vi "Excel - Open Docuement Tests.vi"(8 "error in (no error)":errorcluster) -> (0 "error out":errorcluster)   [LabVIEW 2020]
uses:
  src/LabVIEW NPOI/MS-Excel/MS-Excel.lvclass
  D:/Benjamin/Documents/Perso/Code/WC/LabVIEW_NPOI/src/LabVIEW NPOI/Document/Document.lvclass
  src/LabVIEW NPOI/MS-Excel/Get Workbook.vi
  <vilib>/addons/_JKI Toolkits/Caraya/classes/Assert/Assert Not Error.vi
  <vilib>/addons/_JKI Toolkits/Caraya/classes/Assert/Assert False.vi
  <vilib>/addons/_JKI Toolkits/Caraya/classes/Assert/Assert Error.vi
  <vilib>/addons/_JKI Toolkits/Caraya/classes/Assert/Assert True.vi
  D:/Benjamin/Documents/Perso/Code/WC/LabVIEW_NPOI/lib/NPOI 2.1.1/NPOI.dll
  lib/NPOI 2.1.1/NPOI.dll
  src/LabVIEW NPOI/Document/Document.lvclass
  <vilib>/addons/_JKI Toolkits/Caraya/classes/Test/Test.lvclass
  <vilib>/addons/_JKI Toolkits/Caraya/classes/Assert/Assert.lvclass
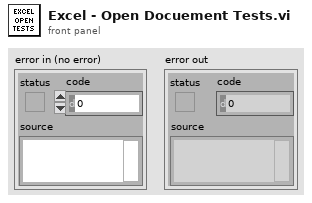
[diagram p1: front panel]
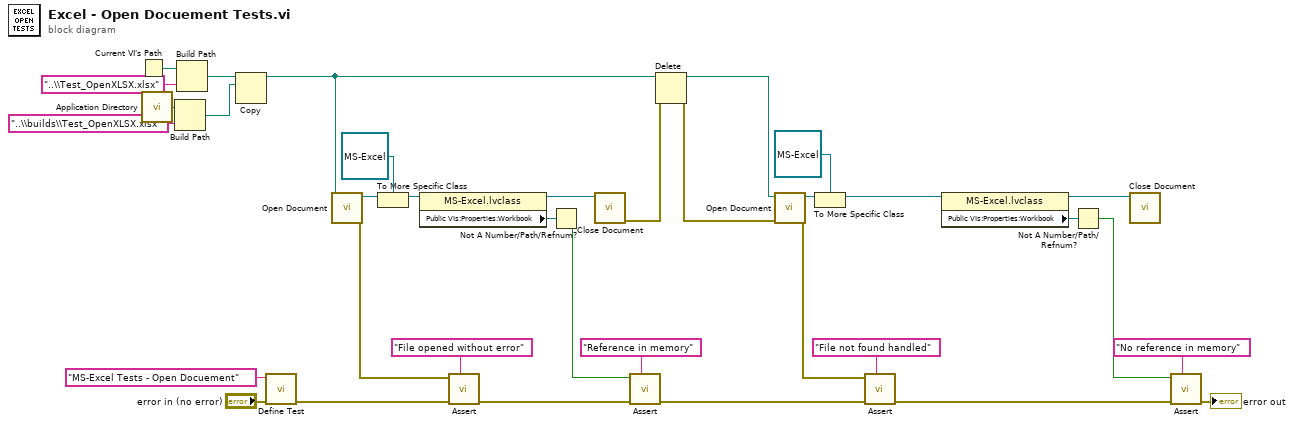
[diagram p0: block diagram]
diagram:
  n1 = Current VI's Path() -> (path=w10:path)
  n2 = call <vilib>:"Application Directory.vi"() -> ("Application Directory"=w12:path)
  n3 = Build Path(base path=w12, name or relative path="..\\builds\\Test_OpenXLSX.xlsx" ("string")) -> (appended path=w7:path)
  n4 = Build Path(base path=w10, name or relative path="..\\Test_OpenXLSX.xlsx" ("string")) -> (appended path=w8:path)
  n5 = Copy(10:w7, 11:w8) -> (3:w6:path)  [unwired: 3 in, 2 out]
  n6 = call <vilib>:"Define Test.vi"("error in (no error)"="error in (no error)", "Label (VI Title)"="MS-Excel Tests - Open Docuement") -> ("error out"=w32:errorcluster)  [unwired: 9 in]
  n7 = call "Open Document.vi"("File Path"=w6) -> ("error out"=w30:errorcluster, "Document out"=w35:refnum<class "Document.lvclass">)  [unwired: 9 in]
  n8 = To More Specific Class(target class=refnum<class "MS-Excel.lvclass"> refnum ("LabVIEW NPOI.lvlib:MS-Excel.lvclass"), reference=w35) -> (specific class reference=w4:refnum<class "MS-Excel.lvclass">)  [unwired: 1 in, 1 out]
  n9 = property class="MS-Excel.lvclass"(reference=w4) -> (reference out=w34:refnum<class "MS-Excel.lvclass">, "Public VIs:Properties:Workbook"=w33:refnum<k24>)  [unwired: 1 in, 1 out]
  n10 = call-poly <vilib>:"Assert.vi"("Label"="File opened without error", "error in (no error)"=w32, "Not Error?"=w30) -> ("error out"=w28:errorcluster)  [unwired: 8 in]
  n11 = Not A Number/Path/Refnum?(number/path/refnum=w33) -> (NaN/Path/Refnum?=w29:bool)
  n12 = call "Close Document.vi"("Document in"=w34) -> ("error out"=w16:errorcluster)  [unwired: 10 in]
  n13 = call-poly <vilib>:"Assert.vi"("Label"="Reference in memory", "error in (no error)"=w28, "False?"=w29) -> ("error out"=w20:errorcluster)  [unwired: 8 in]
  n14 = Delete(path (use dialog)=w6, error in=w16) -> (deleted path=w5:path, error out=w15:errorcluster)  [unwired: 3 in, 1 out]
  n15 = call "Open Document.vi"("error in (no error)"=w15, "File Path"=w5) -> ("error out"=w18:errorcluster, "Document out"=w23:refnum<class "Document.lvclass">)  [unwired: 8 in]
  n16 = To More Specific Class(target class=refnum<class "MS-Excel.lvclass"> refnum ("LabVIEW NPOI.lvlib:MS-Excel.lvclass"), reference=w23) -> (specific class reference=w2:refnum<class "MS-Excel.lvclass">)  [unwired: 1 in, 1 out]
  n17 = call-poly <vilib>:"Assert.vi"("Label"="File not found handled", "error in (no error)"=w20, "Error?"=w18) -> ("error out"=w21:errorcluster)  [unwired: 8 in]
  n18 = property class="MS-Excel.lvclass"(reference=w2) -> (reference out=w24:refnum<class "MS-Excel.lvclass">, "Public VIs:Properties:Workbook"=w25:refnum<k24>)  [unwired: 1 in, 1 out]
  n19 = Not A Number/Path/Refnum?(number/path/refnum=w25) -> (NaN/Path/Refnum?=w17:bool)
  n20 = call "Close Document.vi"("Document in"=w24) -> ()  [unwired: 10 in, 1 out]
  n21 = call-poly <vilib>:"Assert.vi"("Label"="No reference in memory", "error in (no error)"=w21, "True?"=w17) -> ("error out"=→"error out":errorcluster)  [unwired: 8 in]
